vi "Subscribe to Endpoint.vi"(7 "Data Handler":refnum<class "SubscribedDataHandler.lvclass">, 8 "error in (no error)":errorcluster, 10 "Publish Config":T1, 11 "VolatusAPI in":refnum<class "VolatusAPI.lvclass">) -> (0 "error out":errorcluster, 3 "VolatusAPI out":refnum<class "VolatusAPI.lvclass">)   [LabVIEW 2020, in "Volatus.lvlib" / "VolatusAPI.lvclass"]
uses:
  VolatusAPI.lvclass
  VolatusAPI.lvclass/VolatusAPI.ctl
  lv-vecto/Vecto/RemoteDataService/RemoteDataService.lvclass
  lv-vecto/Vecto/Publish Config.ctl
  lv-vecto/VectoConfig/VectoConfig.lvlib
  lv-vecto/Vecto/SubscribedDataHandler/SubscribedDataHandler.lvclass
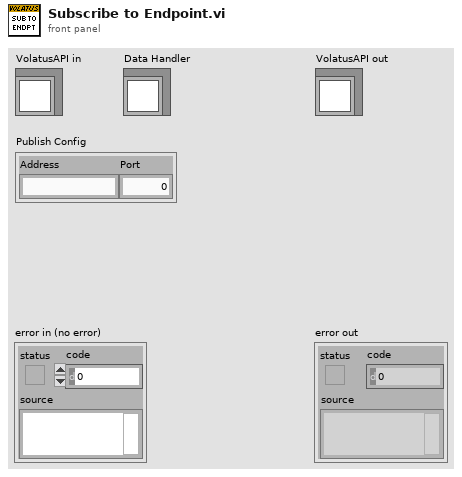
[diagram p1: front panel]
types:
  T1 = typedef "VectoConfig.lvlib/Publish Config.ctl" = cluster{"Address":string, "Port":u16}
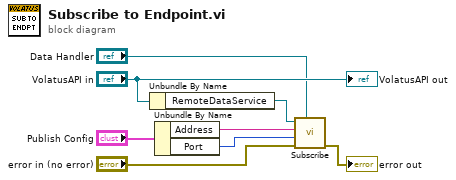
[diagram p0: block diagram]
diagram:
  n1 = Unbundle By Name("VolatusAPI in") -> ("RemoteDataService"=w7:refnum<class "RemoteDataService.lvclass">)
  n2 = Unbundle By Name("Publish Config") -> ("Address"=w3:string, "Port"=w4:u16)
  n3 = call "Subscribe.vi"("DataHandler (None)"="Data Handler", "error in (no error)"="error in (no error)", "Multicast Port"=w4, "Multicast Address"=w3, "RemoteDataService in"=w7) -> ("error out"=→"error out":errorcluster)  [unwired: 5 in, 1 out]
  "VolatusAPI out" <- "VolatusAPI in"
